vi "Send Drone Message.vi"(11 "Message":string) -> ()   [LabVIEW 2014]
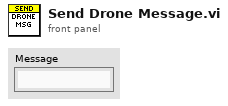
[diagram p1: front panel]
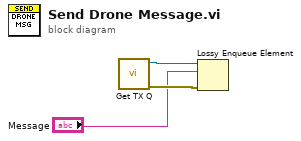
[diagram p0: block diagram]
diagram:
  n1 = call "Get TX Q.vi"() -> ("error out"=w2:errorcluster, "TX Q"=w3:refnum<queue>)  [unwired: 10 in]
  n2 = Lossy Enqueue Element(queue=w3, element="Message", error in (no error)=w2) -> ()  [unwired: 4 out]
